vi "(SubVI) Calculate PSD by ACF or direct FFT.vi"(6 "ACF length":i32=300, 7 "Fs":dbl, 8 "Data":dbl[](array[numeric]), 9 "T=ACF method\nF=direct FT method":bool) -> (0 "df":dbl, 1 "dt":dbl, 2 "PSD":dbl[](array[numeric]), 3 "Frequency,0 df,2df,...,(Hz)":dbl[](array[numeric]))   [LabVIEW 2014]
uses:
  <vilib>/Analysis/2dsp.llb/Real FFT.vi
  <vilib>/Analysis/2dsp.llb/1D Auto Correlation (DBL).vi
  <vilib>/Analysis/NI_AALPro.lvlib
panel:
  out "size(s)":i32
  out "Waveform Graph":dbl[](graph)
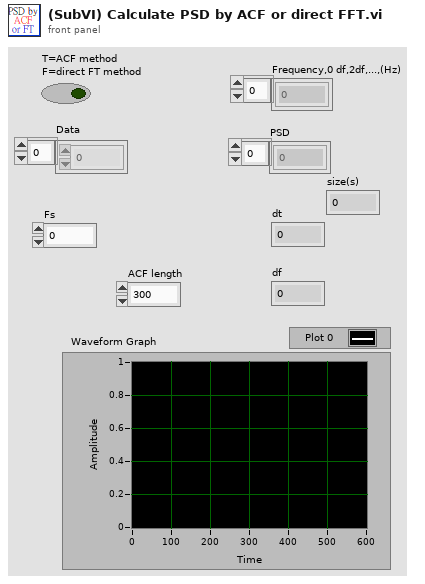
[diagram p1: front panel]
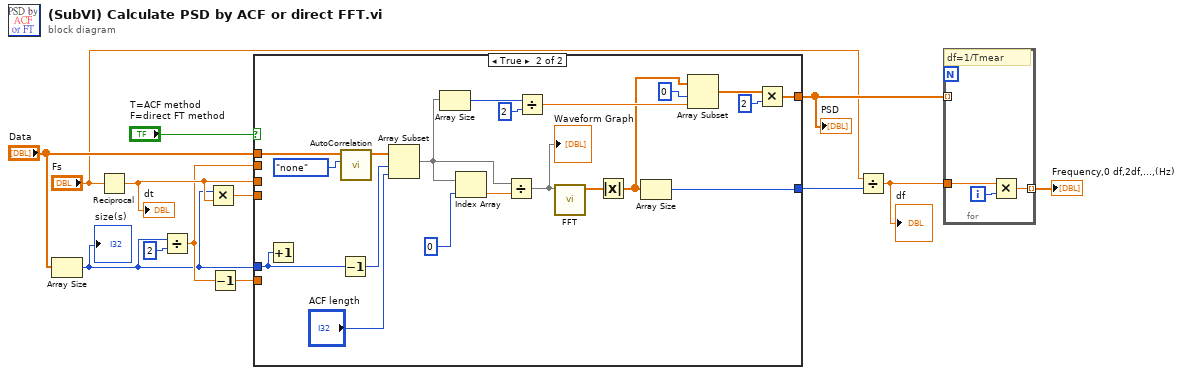
[diagram p0: block diagram]
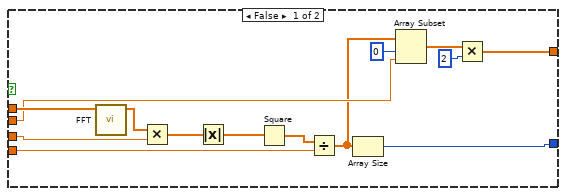
[diagram p2: hidden frame]
diagram:
  n1 = Array Size(array="Data") -> (size(s)=w2:i32)
  "size(s)" <- w2
  n2 = Reciprocal(x="Fs") -> (1/x=w11:dbl)
  "dt" <- w11
  n3 = Divide(x=w2, y=2) -> (x/y=w3:dbl)
  n4 = Multiply(x=w2, y=w11) -> (x*y=w10:dbl)
  n5 = Decrement(x=w3) -> (x-1=w8:dbl)
  n6 = case shown="True" "T=ACF method\nF=direct FT method" {
    tunnel: "Data" -> [w27 w47]
    tunnel: [w17 w41] -> w7
    tunnel: w11 -> [w23 _]
    tunnel: w10 -> [w21 _]
    tunnel: w8 -> [_ _]
    tunnel: w3 -> [w16 _]
    tunnel: w2 -> [_ w35]
    tunnel: [w14 w28] -> w1
    frame False {
      n7 = call-poly <vilib>:"FFT.vi"("X"=w27) -> ("FFT {X}"=w24:cdb[])  [unwired: 9 in, 1 out]
      n8 = Multiply(x=w24, y=w23) -> (x*y=w22:cdb[])
      n9 = Absolute Value(x=w22) -> (abs(x)=w26:dbl[])
      n10 = Square(x=w26) -> (x^2=w25:dbl[])
      n11 = Divide(x=w25, y=w21) -> (x/y=w15:dbl[])
      n12 = Array Size(array=w15) -> (size(s)=w14:i32)
      n13 = Array Subset(array=w15, index=0 ("y"), length=w16) -> (w19:dbl[])
      n14 = Multiply(x=w19, y=2) -> (x*y=w17:dbl[])
    }
    frame True {
      n15 = Increment(x=w35) -> ()  [unwired: 1 out]
      n16 = Decrement(x=w35) -> (x-1=w39:i32)
      n17 = call-poly <vilib>:"AutoCorrelation.vi"("normalization"=enum32{"none", "unbiased", "biased"}."none", "X"=w47) -> ("Rxx"=w40:dbl[])  [unwired: 8 in, 1 out]
      n18 = Array Subset(array=w40, index=w39, length="ACF length") -> (w33:dbl[])
      n19 = Array Size(array=w33) -> (size(s)=w32:i32)
      n20 = Index Array(array=w33, index=0) -> (element=w37:dbl)
      n21 = Divide(x=w33, y=w37) -> (x/y=w36:dbl[])
      "Waveform Graph" <- w36
      n22 = Divide(x=w32, y=2 ("size(s)")) -> (x/y=w30:dbl)
      n23 = call-poly <vilib>:"FFT.vi"("X"=w36) -> ("FFT {X}"=w46:cdb[])  [unwired: 9 in, 1 out]
      n24 = Absolute Value(x=w46) -> (abs(x)=w29:dbl[])
      n25 = Array Size(array=w29) -> (size(s)=w28:i32)
      n26 = Array Subset(array=w29, index=0, length=w30) -> (w43:dbl[])
      n27 = Multiply(x=w43, y=2) -> (x*y=w41:dbl[])
    }
  }
  "PSD" <- w7
  n28 = Divide(x="Fs", y=w1) -> (x/y=w5:dbl)
  "df" <- w5
  n29 = for {
    tunnel: w7 -> [_] mode=indexing
    tunnel: w5 -> [w50]
    tunnel: [w48] -> w4 mode=indexing
    i -> [w49]
    # "df=1/Tmear"
    n30 = Multiply(x=w50, y=w49) -> (x*y=w48:dbl)
  }
  "Frequency,0 df,2df,...,(Hz)" <- w4
